vi "LabVIEWDemo.vi"() -> ()   [LabVIEW 2017]
uses:
  C:/Program Files (x86)/Wasatch Photonics/Wasatch.NET/WasatchNET.dll
panel:
  out "Driver Version":string
  out "FPGA FW":string
  out "microcontroller FW":string
  in  "Trigger":bool
  in  "Fire Laser":bool
  in  "Detector Setpoint (°C)":sgl min=15 max=20
  out "Detector TEC (°C)":dbl format="%.2f"
  out "Serial":string
  out "Model":string
  in  "Integration Time (ms)":u32=100 min=10 max=5000 step=1
  out "Excitation (nm)":dbl
  out "Coeff3":dbl
  out "Coeff2":dbl
  out "Coeff1":dbl
  out "Coeff0":dbl
  in  "Start/Stop":bool
  out "XY Graph":T1(graph)
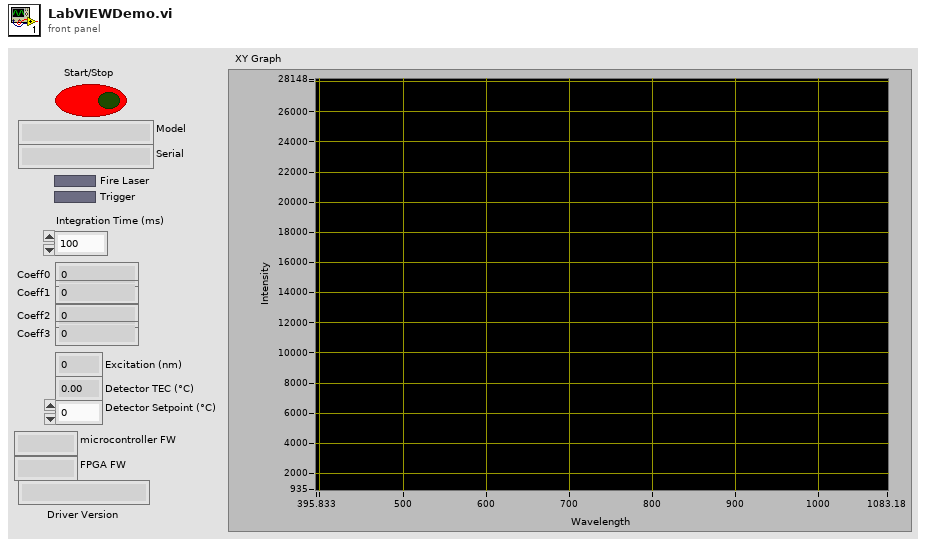
[diagram p1: front panel]
types:
  T1 = cluster{"getSpectrum":dbl[], "wavenumbers":dbl[]}
  T2 = cluster{"wavelengths":dbl[], "getSpectrum":dbl[]}
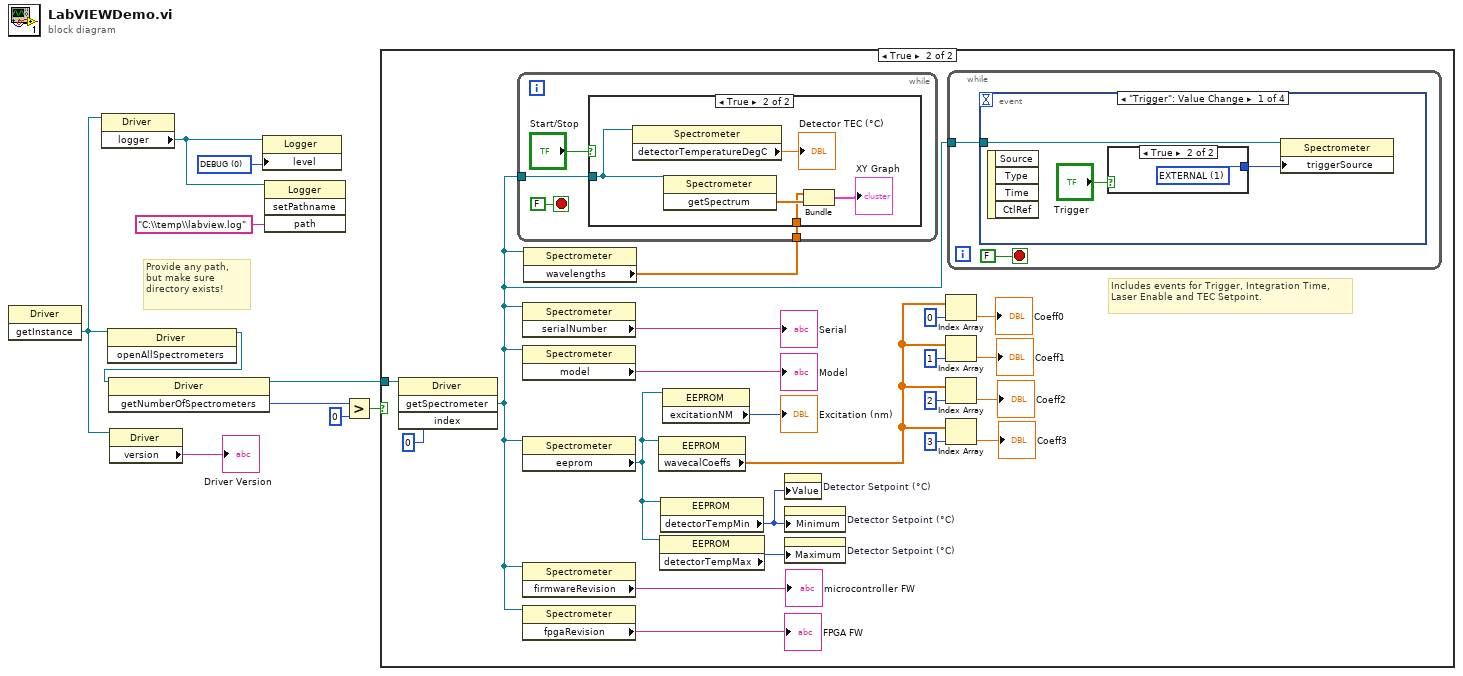
[diagram p0: block diagram]
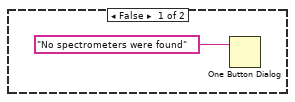
[diagram p2: hidden frame]
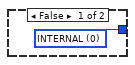
[diagram p3: hidden frame]
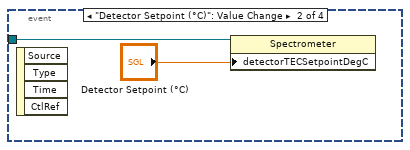
[diagram p4: hidden frame]
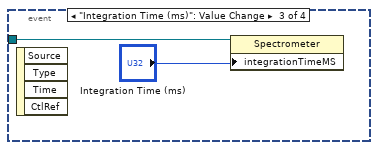
[diagram p5: hidden frame]
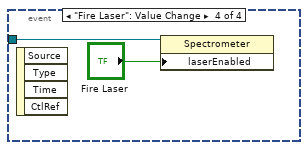
[diagram p6: hidden frame]
diagram:
  w9 = 0 items=["DEBUG", "INFO", "ERROR", "NEVER"] ("level")
  # "Provide any path,\nbut make sure\ndirectory exists!"
  n1 = invoke on="Invoke Node" class="Driver" method="getInstance"() -> ("getInstance"=w3:refnum<k24>)  [unwired: 3 in, 2 out]
  n2 = property class="Driver"(reference=w3) -> ("logger"=w1:refnum<k24>)  [unwired: 1 in, 2 out]
  n3 = invoke class="Driver" method="openAllSpectrometers"(reference=w3) -> (reference out=w2:refnum<k24>)  [unwired: 2 in, 2 out]
  n4 = invoke class="Driver" method="getNumberOfSpectrometers"(reference=w2) -> (reference out=w5:refnum<k24>, "getNumberOfSpectrometers"=w8:i32)  [unwired: 2 in, 1 out]
  n5 = property class="Driver"(reference=w3) -> ("version"=→"Driver Version":string)  [unwired: 1 in, 2 out]
  n6 = property class="Logger"(reference=w1, "level"=w9) -> ()  [unwired: 1 in, 2 out]
  n7 = invoke class="Logger" method="setPathname"(reference=w1, "path"="C:\\temp\\labview.log") -> ()  [unwired: 2 in, 4 out]
  n8 = Greater?(x=w8, y=0) -> (0:w6:bool)
  n9 = case shown="True" w6 {
    tunnel: w5 -> [_ w16]
    frame False {
      n10 = One Button Dialog(message="No spectrometers were found") -> ()  [unwired: 1 in, 1 out]
    }
    frame True {
      # "Includes events for Trigger, Integration Time, Laser Enable and TEC Setpoint."
      n11 = invoke on="Invoke Node" class="Driver" method="getSpectrometer"(reference=w16, "index"=0) -> ("getSpectrometer"=w12:refnum<k24>)  [unwired: 2 in, 3 out]
      n12 = property class="Spectrometer"(reference=w12) -> ("serialNumber"=→"Serial":string)  [unwired: 1 in, 2 out]
      n13 = property class="Spectrometer"(reference=w12) -> ("model"=→"Model":string)  [unwired: 1 in, 2 out]
      n14 = property class="Spectrometer"(reference=w12) -> ("eeprom"=w31:refnum<k24>)  [unwired: 1 in, 2 out]
      n15 = property class="Spectrometer"(reference=w12) -> ("firmwareRevision"=→"microcontroller FW":string)  [unwired: 1 in, 2 out]
      n16 = property class="Spectrometer"(reference=w12) -> ("fpgaRevision"=→"FPGA FW":string)  [unwired: 1 in, 2 out]
      n17 = property class="Spectrometer"(reference=w12) -> ("wavelengths"=w13:dbl[])  [unwired: 1 in, 2 out]
      n18 = while {
        tunnel: w12 -> [w48]
        tunnel: w13 -> [w46]
        stop <- FALSE stop-if-true
        n19 = case shown="True" "Start/Stop" {
          tunnel: w48 -> [_ w51]
          tunnel: w46 -> [_ w50]
          frame False {
          }
          frame True {
            n20 = property class="Spectrometer"(reference=w51) -> ("detectorTemperatureDegC"=→"Detector TEC (°C)":sgl)  [unwired: 1 in, 2 out]
            n21 = invoke class="Spectrometer" method="getSpectrum"(reference=w51) -> ("getSpectrum"=w54:dbl[])  [unwired: 2 in, 2 out]
            n22 = Bundle("wavelengths"=w50, "getSpectrum"=w54) -> (→"XY Graph":T2)  [unwired: 1 in]
          }
        }
      }
      n23 = property class="EEPROM"(reference=w31) -> ("wavecalCoeffs"=w23:sgl[])  [unwired: 1 in, 2 out]
      n24 = property class="EEPROM"(reference=w31) -> ("detectorTempMax"=w30:i16)  [unwired: 1 in, 2 out]
      n25 = property class="EEPROM"(reference=w31) -> ("detectorTempMin"=w32:i16)  [unwired: 1 in, 2 out]
      n26 = property class="EEPROM"(reference=w31) -> ("excitationNM"=→"Excitation (nm)":u16)  [unwired: 1 in, 2 out]
      n27 = property on="Detector Setpoint (°C)" class="DigNum (strict)"("Value"=w32) -> ()  [unwired: 2 in, 2 out]
      n28 = property on="Detector Setpoint (°C)" class="DigNum (strict)"("Minimum"=w32) -> ()  [unwired: 2 in, 2 out]
      n29 = property on="Detector Setpoint (°C)" class="DigNum (strict)"("Maximum"=w30) -> ()  [unwired: 2 in, 2 out]
      n30 = Index Array(array=w23, index=0) -> (element=→"Coeff0":sgl)
      n31 = Index Array(array=w23, index=1 ("1")) -> (element=→"Coeff1":sgl)
      n32 = Index Array(array=w23, index=2) -> (element=→"Coeff2":sgl)
      n33 = Index Array(array=w23, index=3) -> (element=→"Coeff3":sgl)
      n34 = while {
        tunnel: w12 -> [w34]
        stop <- FALSE stop-if-true
        n35 = event shown="[0] \"Trigger\": Value Change" {
          selector: _ -> [_ _ _ _]
          dyn-events: _ -> [_ _ _ _]
          timeout: _ -> [_ _ _ _]
          tunnel: w34 -> [w37 w41 w43 w45]
          event "Trigger": Value Change {
            n36 = event-data() -> ()  [unwired: 1 in, 4 out]
            n37 = case shown="True" "Trigger" {
              tunnel: [w38 w39] -> w36
              frame False {
                w38 = 0 items=["INTERNAL", "EXTERNAL", "ERROR"] ("triggerSource")
              }
              frame True {
                w39 = 1 items=["INTERNAL", "EXTERNAL", "ERROR"] ("triggerSource")
              }
            }
            n38 = property class="Spectrometer"(reference=w37, "triggerSource"=w36) -> ()  [unwired: 1 in, 2 out]
          }
          event "Detector Setpoint (°C)": Value Change {
            n39 = event-data() -> ()  [unwired: 1 in, 4 out]
            n40 = property class="Spectrometer"(reference=w41, "detectorTECSetpointDegC"="Detector Setpoint (°C)") -> ()  [unwired: 1 in, 2 out]
          }
          event "Integration Time (ms)": Value Change {
            n41 = event-data() -> ()  [unwired: 1 in, 4 out]
            n42 = property class="Spectrometer"(reference=w43, "integrationTimeMS"="Integration Time (ms)") -> ()  [unwired: 1 in, 2 out]
          }
          event "Fire Laser": Value Change {
            n43 = event-data() -> ()  [unwired: 1 in, 4 out]
            n44 = property class="Spectrometer"(reference=w45, "laserEnabled"="Fire Laser") -> ()  [unwired: 1 in, 2 out]
          }
        }
      }
    }
  }
